vi "Save Configuration Settings to XML.vi"(8 "error in (no error)":errorcluster, 11 "User Configuration":T1={"Hardware Configuration"={"Signal Channel"="", "Response Channel"="", "Trigger Channel"="", "Number of acquisitions"=0.0}, "Analysis Configuration"={"Statistics"=TRUE}, "Signal Type"=enum."Single Chirp", "New Data Behavior"=enum."Replace", "Signal Configuration"={"Chirp Amplitude"=0.1, "I/O Limit"=10.0, "Sample Rate"=1000000.0, "Chirp Duration (s)"=10000000.0, "Upper Frequency"=0.0, "Lower Frequency"=0.0, "Windowing"=enum."None"}}) -> (0 "error out":errorcluster)   [LabVIEW 2017]
doc: "Saves the user-specified configuration data to an XML file. This is used to remember settings between executions."
uses:
  controls/User Specified Data.ctl
  controls/HW Configuration.ctl
  controls/Analysis Configuration.ctl
  controls/New Data Behavior.ctl
  controls/Signal Configuration.ctl
  <vilib>/Utility/xml.llb/Write to XML File(string).vi
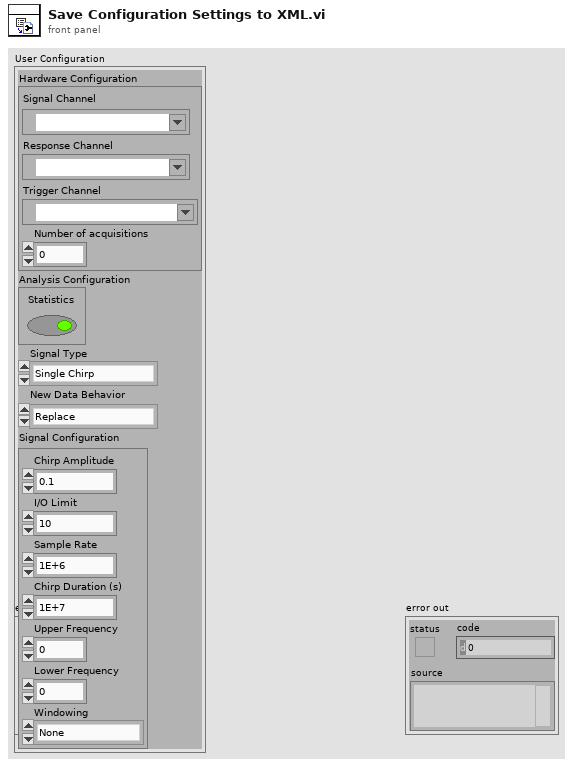
[diagram p1: front panel]
types:
  T1 = typedef "User Specified Data.ctl" = cluster{"Hardware Configuration":T2, "Analysis Configuration":T3, "Signal Type":enum16{"Single Chirp", "From Excel"}, "New Data Behavior":T4, "Signal Configuration":T5}
  T2 = typedef "HW Configuration.ctl" = cluster{"Signal Channel":tag, "Response Channel":tag, "Trigger Channel":tag, "Number of acquisitions":dbl}
  T3 = typedef "Analysis Configuration.ctl" = cluster{"Statistics":bool}
  T4 = typedef "New Data Behavior.ctl" = enum16{"Replace", "Overlay", "Append"}
  T5 = typedef "Signal Configuration.ctl" = cluster{"Chirp Amplitude":dbl, "I/O Limit":dbl, "Sample Rate":dbl, "Chirp Duration (s)":dbl, "Upper Frequency":dbl, "Lower Frequency":dbl, "Windowing":enum16{"None", "Exponential", "Flat top", "Hamming", "Hanning", "Kaiser-Bessel", "Rectangular"}}
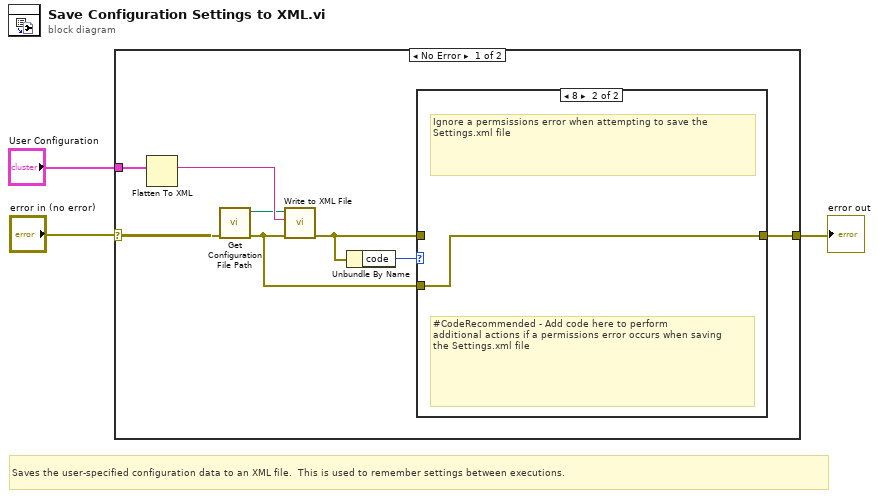
[diagram p0: block diagram]
diagram:
  # "Saves the user-specified configuration data to an XML file.  This is used to remember settings between executions."
  n1 = case shown="No Error" "error in (no error)" {
    selector: "error in (no error)" -> [w8 w14]
    tunnel: [w5 w14] -> w2
    tunnel: "User Configuration" -> [w11 _]
    frame No Error {
      n2 = Flatten To XML(anything=w11) -> (xml string=w10:string)
      n3 = call "Get Configuration File Path.vi"("error in (no error)"=w8) -> ("error out"=w4:errorcluster, "XML File Path"=w9:path)  [unwired: 9 in]
      n4 = call-poly <vilib>:"Write to XML File.vi"("error in (no error)"=w4, "XML Input"=w10, "XML File Path"=w9) -> ("error out"=w6:errorcluster)  [unwired: 6 in, 2 out]
      n5 = Unbundle By Name(w6) -> ("code"=w7:i32)
      n6 = case shown="8" w7 {
        tunnel: w6 -> [w12 _]
        tunnel: [w12 w13] -> w5
        tunnel: w4 -> [_ w13]
        frame Default {
        }
        frame 8 {
          # "#CodeRecommended - Add code here to perform\nadditional actions if a permissions error occurs when saving\nthe Settings.xml file"
          # "Ignore a permsissions error when attempting to save the\nSettings.xml file"
        }
      }
    }
    frame Error {
    }
  }
  "error out" <- w2
